vi "LAVA.move picture.vi"(10 "Picture in":picture, 11 "background":picture) -> (2 "Picture out":picture)   [LabVIEW 2021, in "Pop-Up.lvlib" / "Popup.lvclass"]
doc: "adapted from: https://lavag.org/topic/17138-2d-picture-translation-movement/#comment-105597"
uses:
  Popup.lvclass
  Popup.lvclass/Popup.ctl
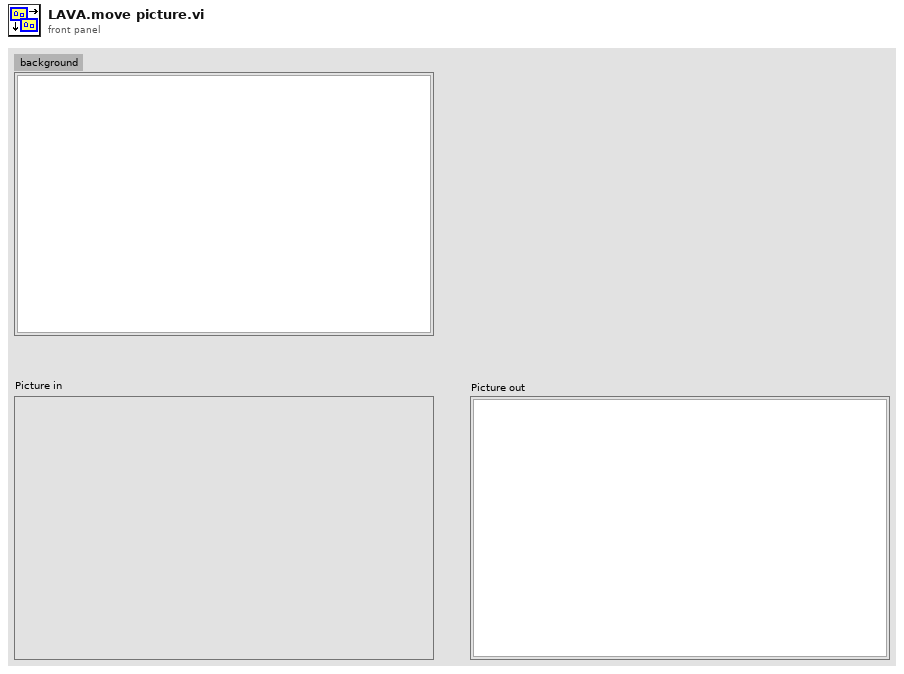
[diagram p1: front panel]
types:
  T1 = typedef "Pop-Up.lvlib/Popup.lvclass/LAVA.picture op-code.ctl" = u16
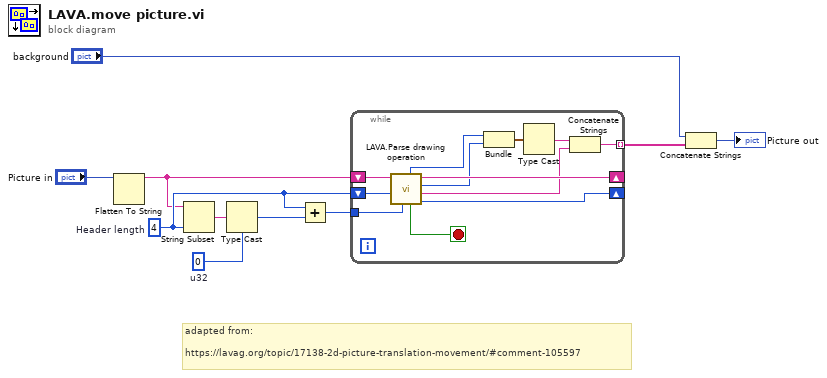
[diagram p0: block diagram]
diagram:
  w2 = u32 0  # u32
  w9 = 4  # Header length
  # "adapted from: \n\nhttps://lavag.org/topic/17138-2d-picture-translation-movement/#comment-105597"
  n1 = Flatten To String(anything="Picture in") -> (data string=w4:string)  [unwired: 3 in, 2 out]
  n2 = String Subset(string=w4, length (rest)=w9) -> (substring=w3:string)  [unwired: 1 in]
  n3 = Type Cast(type=w2, x=w3) -> (*(type *) &x=w10:u32)
  n4 = Add(x=w9, y=w10) -> (x+y=w8:u32)
  n5 = while {
    shift-right: [w17] -> _
    shift-left: w4 -> [w21]
    shift-right: [w20] -> _
    shift-left: w9 -> [w22]
    tunnel: w8 -> [w18]
    tunnel: [w13] -> w6 mode=indexing
    stop <- w19 stop-if-true
    n6 = call "LAVA.Parse drawing operation.vi"("picture size"=w18, "offset"=w22, "picture data in"=w21) -> ("offset past element"=w20:i32, "data string"=w12:string, "data length"=w16:u32, "picture data out"=w17:string, "last element"=w19:bool, "op-code"=w11:T1)  [unwired: 3 in]
    n7 = Bundle("op-code"=w11, "data length"=w16) -> (w15:cluster{"op-code":T1, "data length":u32})  [unwired: 1 in]
    n8 = Type Cast(x=w15) -> (*(type *) &x=w14:string)  [unwired: 1 in]
    n9 = Concatenate Strings(w14, w12) -> (w13:string)
  }
  n10 = Concatenate Strings("background", w6) -> (→"Picture out":picture)
